vi "Calibration Caluclation(SubVI).vi"(6 "reference in":refnum<vi>, 9 "reference 3":refnum<vi>, 10 "reference 4":refnum<vi>, 11 "Digital in":refnum<vi>) -> (2 "Y intercept":dbl, 3 "Gradient":dbl)   [LabVIEW 2011]
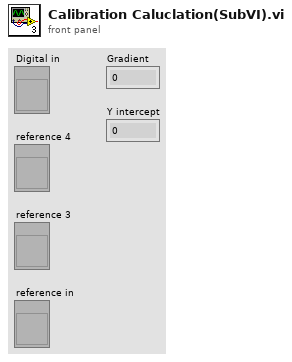
[diagram p1: front panel]
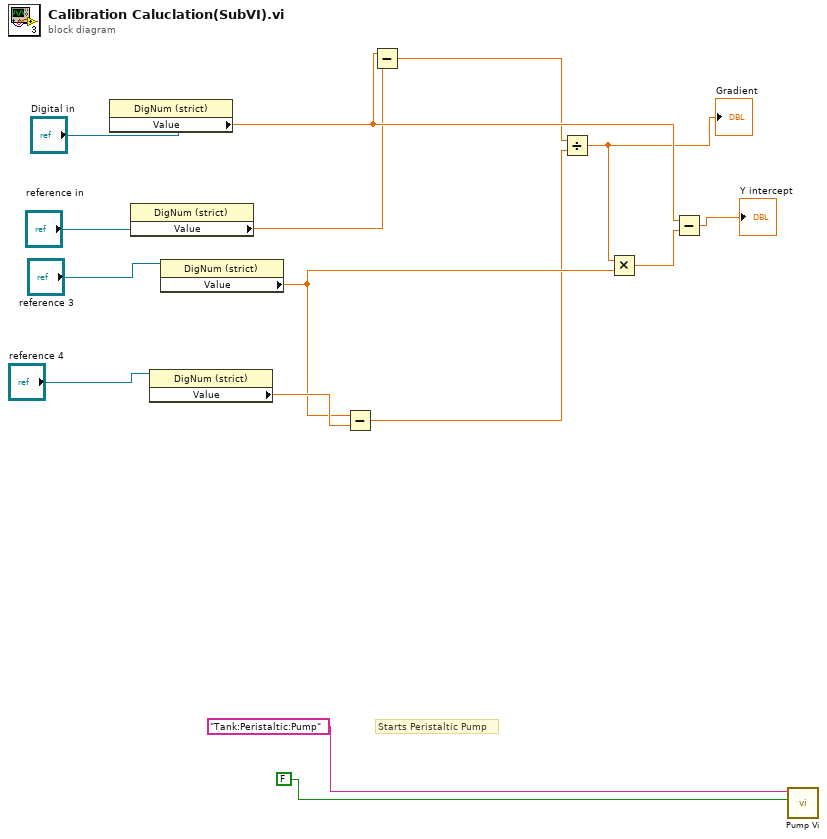
[diagram p0: block diagram]
diagram:
  # "Starts Peristaltic Pump"
  n1 = property class="DigNum (strict)"(reference="Digital in") -> ("Value"=w15:dbl)  [unwired: 1 in, 2 out]
  n2 = property class="DigNum (strict)"(reference="reference in") -> ("Value"=w10:dbl)  [unwired: 1 in, 2 out]
  n3 = property class="DigNum (strict)"(reference="reference 4") -> ("Value"=w14:dbl)  [unwired: 1 in, 2 out]
  n4 = property class="DigNum (strict)"(reference="reference 3") -> ("Value"=w13:dbl)  [unwired: 1 in, 2 out]
  n5 = Subtract(x=w13, y=w14) -> (x-y=w12:dbl)
  n6 = Subtract(x=w15, y=w10) -> (x-y=w11:dbl)
  n7 = Divide(x=w11, y=w12) -> (x/y=w5:dbl)
  "Gradient" <- w5
  n8 = Multiply(x=w5, y=w13) -> (x*y=w6:dbl)
  n9 = Subtract(x=w15, y=w6) -> (x-y=→"Y intercept":dbl)
  n10 = call "Pump Vi.vi"("Boolean"=FALSE, "Channel Name"="Tank:Peristaltic:Pump") -> ()  [unwired: 8 in, 2 out]
